vi "sub build sound.vi"(8 "error in":errorcluster, 11 "sound":string) -> (0 "error out":errorcluster, 3 "sound string":string)   [LabVIEW 2018, in "Frame Analizer.lvclass"]
uses:
  Frame Analizer.lvclass
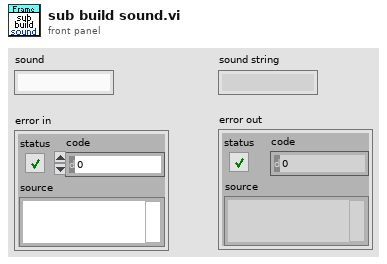
[diagram p1: front panel]
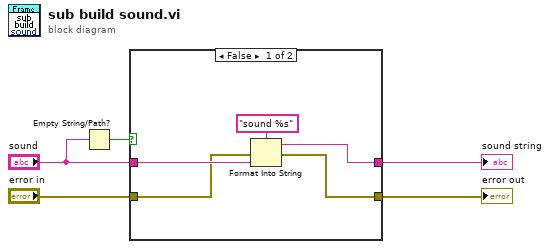
[diagram p0: block diagram]
diagram:
  n1 = Empty String/Path?(string/path="sound") -> (empty?=w1:bool)
  n2 = case shown="False" w1 {
    tunnel: "sound" -> [w10 _]
    tunnel: "error in" -> [w8 w11]
    tunnel: [w7 w11] -> w3
    tunnel: [w6 _] -> w2
    frame False {
      n3 = Format Into String(format string="sound %s", error in=w8, w10) -> (resulting string=w6:string, error out=w7:errorcluster)  [unwired: 1 in]
    }
    frame True {
    }
  }
  "sound string" <- w2
  "error out" <- w3
